vi "InterpClamped.vi"(8 "x value":dbl format="%0.2f", 10 "X":dbl[](array[numeric]) format="%0.2f", 11 "Y":dbl[](array[numeric]) format="%0.2f") -> (0 "unclamped value":dbl format="%0.2f", 3 "clamped value":dbl format="%0.2f")   [LabVIEW 2013]
doc: "Performs polynomial interpolation with values clamped to the endpoints."
uses:
  <vilib>/Analysis/NI_AALPro.lvlib
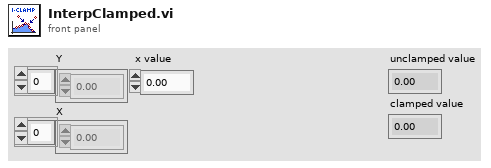
[diagram p1: front panel]
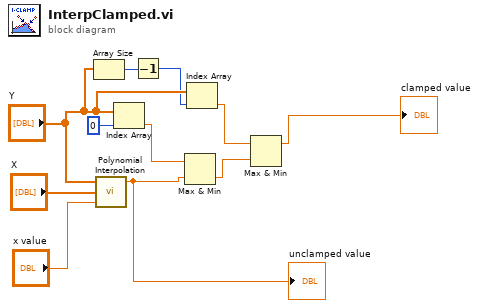
[diagram p0: block diagram]
diagram:
  n1 = Array Size(array="Y") -> (size(s)=w2:i32)
  n2 = call <vilib>:"Polynomial Interpolation.vi"("x value"="x value", "X"="X", "Y"="Y") -> ("interpolation value"=w8:dbl)  [unwired: 2 out]
  "unclamped value" <- w8
  n3 = Index Array(array="Y", index=0) -> (element=w9:dbl)
  n4 = Decrement(x=w2) -> (x-1=w1:i32)
  n5 = Max & Min(x=w9, y=w8) -> (min(x,y)=w4:dbl)  [unwired: 1 out]
  n6 = Index Array(array="Y", index=w1) -> (element=w5:dbl)
  n7 = Max & Min(x=w5, y=w4) -> (max(x,y)=→"clamped value":dbl)  [unwired: 1 out]
